vi "FlashAll.vi"(8 "error in":errorcluster caption="错误输入", 11 "Setup":T3) -> (0 "error out":errorcluster caption="错误输出", 2 "参数配置":T1, 3 "型号参数":T2)   [LabVIEW 2013]
uses:
  SetupCtl.ctl
  Model.ctl
  ParaConfig.ctl
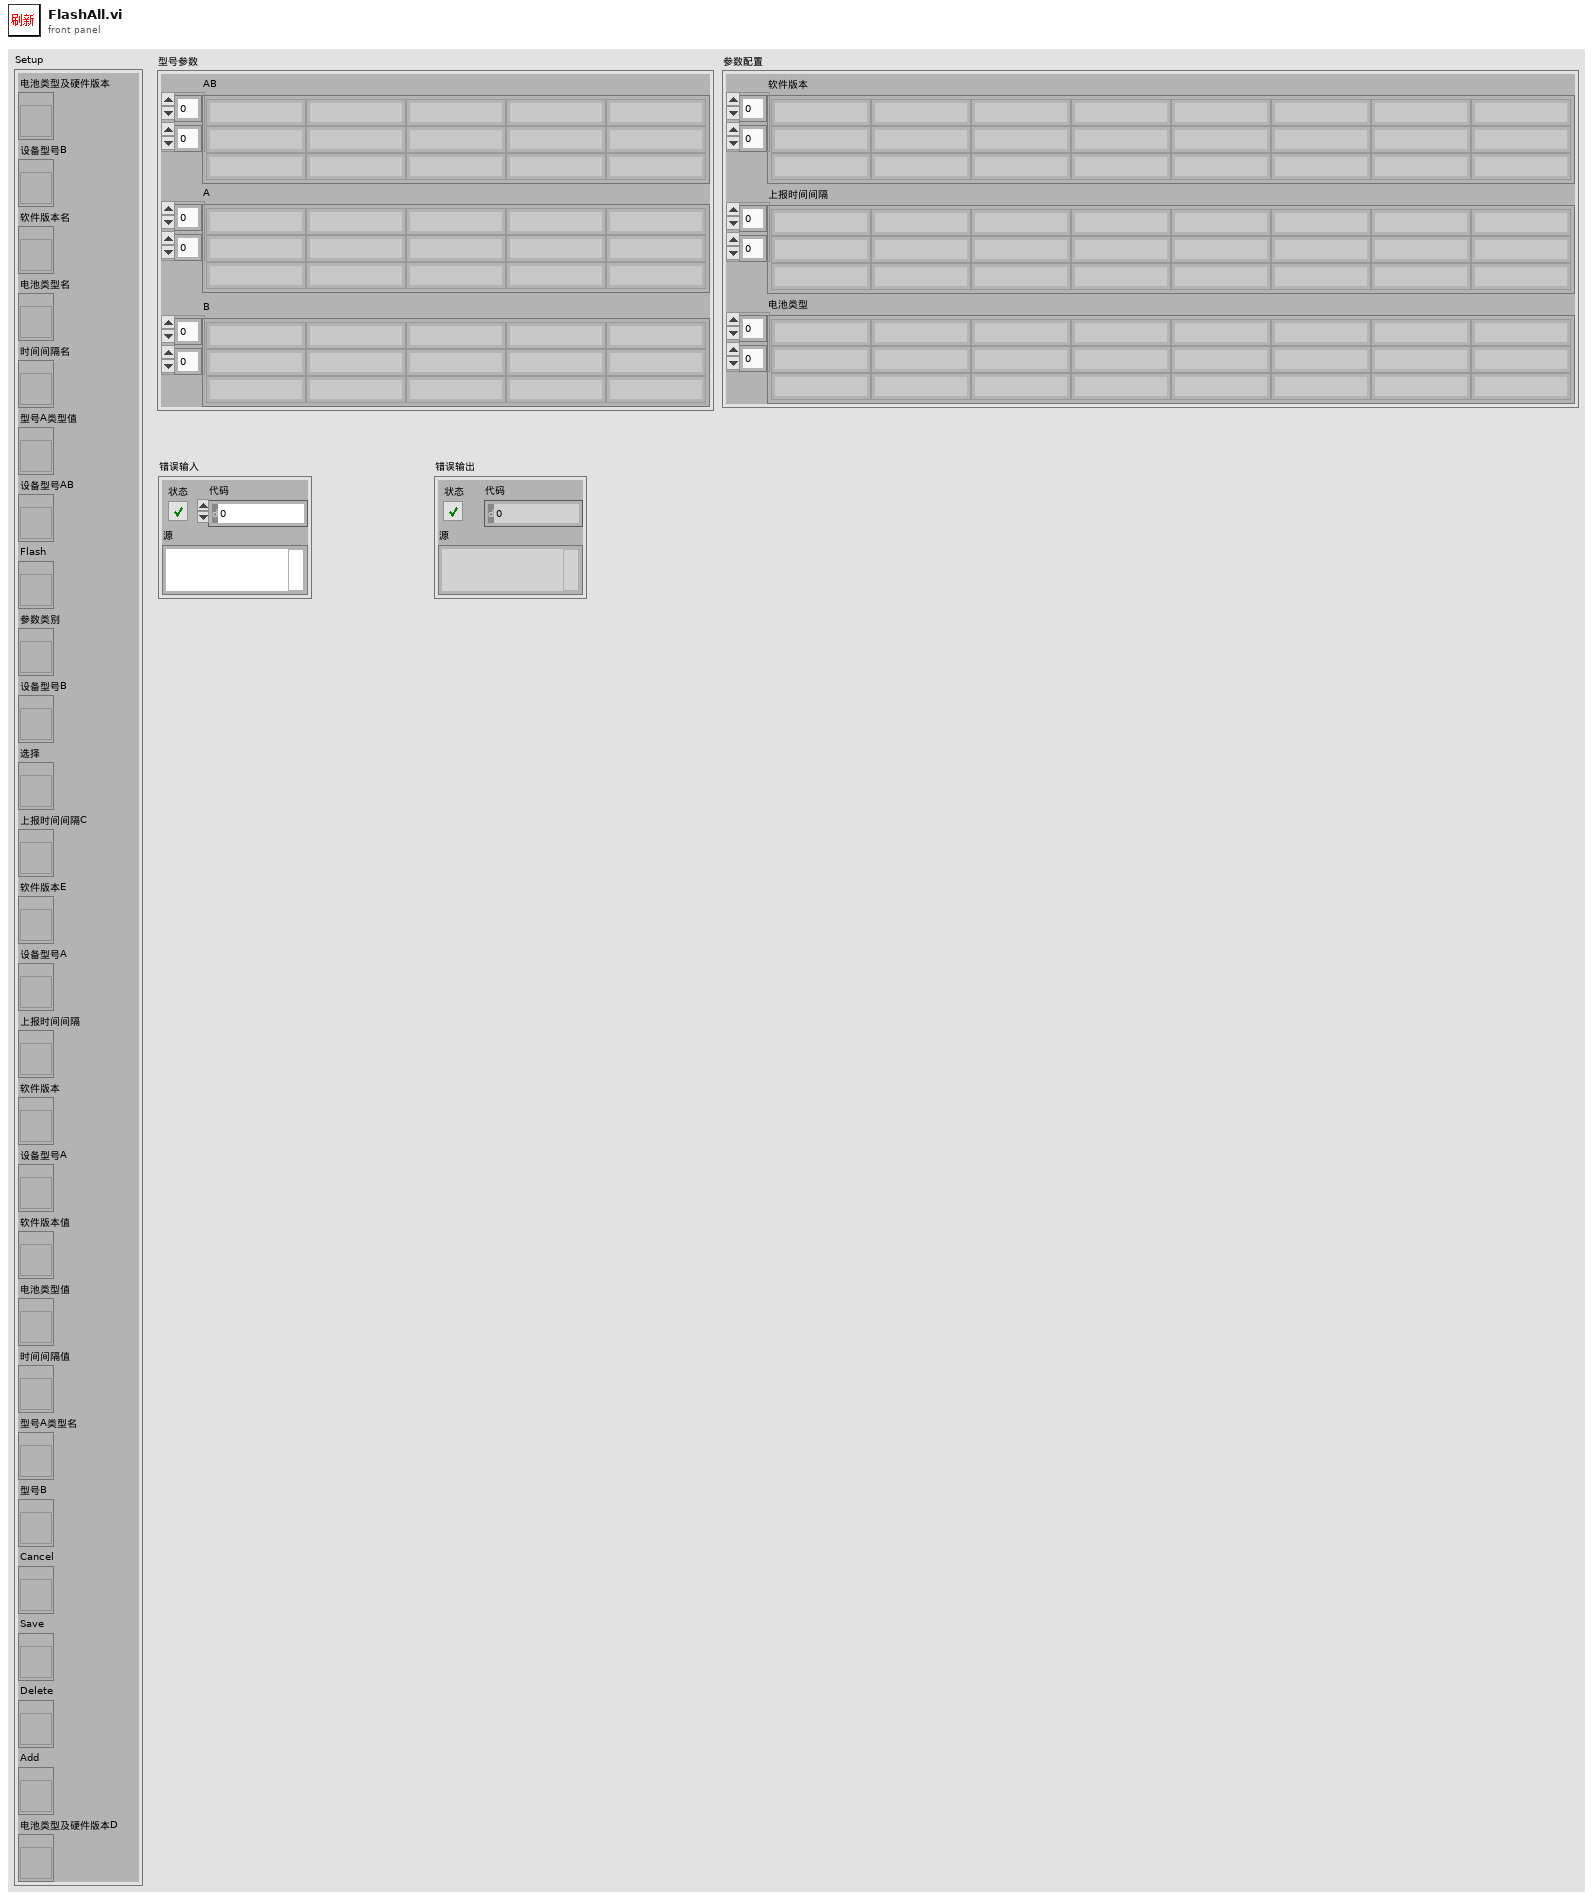
[diagram p1: front panel]
types:
  T1 = typedef "ParaConfig.ctl" = cluster{"软件版本":string[][], "上报时间间隔":string[][], "电池类型":string[][]}
  T2 = typedef "Model.ctl" = cluster{"AB":string[][], "A":string[][], "B":string[][]}
  T3 = typedef "SetupCtl.ctl" = cluster{"电池类型及硬件版本":refnum<vi>, "设备型号B":refnum<vi>, "软件版本名":refnum<vi>, "电池类型名":refnum<vi>, "时间间隔名":refnum<vi>, "型号A类型值":refnum<vi>, "设备型号AB":refnum<vi>, "Flash":refnum<vi>, "参数类别":refnum<vi>, "设备型号B":refnum<vi>, "选择":refnum<vi>, "上报时间间隔C":refnum<vi>, "软件版本E":refnum<vi>, "设备型号A":refnum<vi>, "上报时间间隔":refnum<vi>, "软件版本":refnum<vi>, "设备型号A":refnum<vi>, "软件版本值":refnum<vi>, "电池类型值":refnum<vi>, "时间间隔值":refnum<vi>, "型号A类型名":refnum<vi>, "型号B":refnum<vi>, "Cancel":refnum<vi>, "Save":refnum<vi>, "Delete":refnum<vi>, "Add":refnum<vi>, "电池类型及硬件版本D":refnum<vi>}
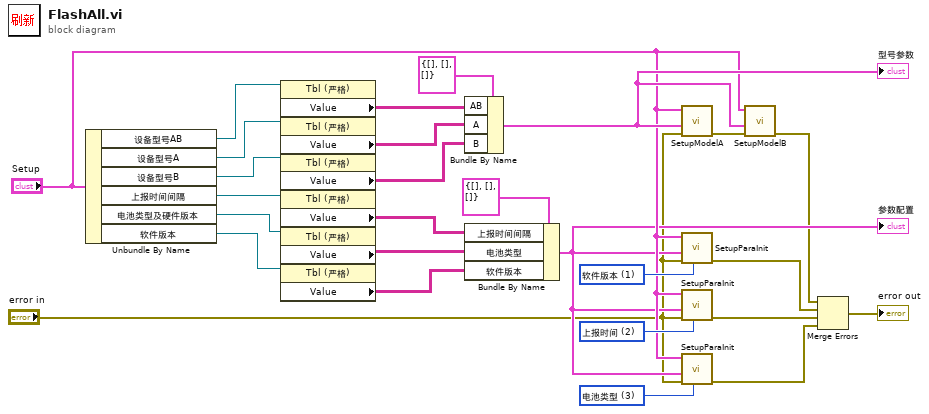
[diagram p0: block diagram]
diagram:
  w7 = u16 3 items=["软件版本"=1, "上报时间"=2, "电池类型"=3] ("参数选择")
  w10 = u16 2 items=["软件版本"=1, "上报时间"=2, "电池类型"=3] ("参数选择")
  w11 = u16 1 items=["软件版本"=1, "上报时间"=2, "电池类型"=3] ("参数选择")
  n1 = Unbundle By Name("Setup") -> ("设备型号AB"=w25:refnum<vi>, "设备型号A"=w24:refnum<vi>, "设备型号B"=w23:refnum<vi>, "上报时间间隔"=w22:refnum<vi>, "电池类型及硬件版本"=w21:refnum<vi>, "软件版本"=w20:refnum<vi>)
  n2 = property class="Tbl (严格)"(reference=w25) -> ("Value"=w19:string[][])  [unwired: 1 in, 2 out]
  n3 = property class="Tbl (严格)"(reference=w24) -> ("Value"=w18:string[][])  [unwired: 1 in, 2 out]
  n4 = property class="Tbl (严格)"(reference=w23) -> ("Value"=w17:string[][])  [unwired: 1 in, 2 out]
  n5 = property class="Tbl (严格)"(reference=w22) -> ("Value"=w16:string[][])  [unwired: 1 in, 2 out]
  n6 = property class="Tbl (严格)"(reference=w21) -> ("Value"=w15:string[][])  [unwired: 1 in, 2 out]
  n7 = property class="Tbl (严格)"(reference=w20) -> ("Value"=w14:string[][])  [unwired: 1 in, 2 out]
  n8 = Bundle By Name(cluster=T2 {"AB"=[], "A"=[], "B"=[]} ("设备型号AB"), "AB"=w19, "A"=w18, "B"=w17) -> (w12:T2)
  "型号参数" <- w12
  n9 = Bundle By Name(cluster=T1 {"软件版本"=[], "上报时间间隔"=[], "电池类型"=[]} ("参数配置"), "上报时间间隔"=w16, "电池类型"=w15, "软件版本"=w14) -> (w8:T1)
  "参数配置" <- w8
  n10 = call "SetupModelA.vi"("error in"="error in", "设备型号AB"=w12, "Setup"="Setup") -> ("error out"=w13:errorcluster)  [unwired: 8 in]
  n11 = call "SetupParaInit.vi"("参数选择"=w11, "error in"="error in", "参数配置"=w8, "Setup"="Setup") -> ("error out"=w4:errorcluster)  [unwired: 7 in]
  n12 = call "SetupParaInit.vi"("参数选择"=w10, "error in"="error in", "参数配置"=w8, "Setup"="Setup") -> ("error out"=w3:errorcluster)  [unwired: 7 in]
  n13 = call "SetupParaInit.vi"("参数选择"=w7, "error in"="error in", "参数配置"=w8, "Setup"="Setup") -> ("error out"=w2:errorcluster)  [unwired: 7 in]
  n14 = call "SetupModelB.vi"("error in"=w13, "设备型号AB"=w12, "Setup"="Setup") -> ("error out"=w5:errorcluster)  [unwired: 8 in]
  n15 = Merge Errors(w5, w4, w3, w2) -> (→"error out":errorcluster)
